vi "ASCII表.vi"() -> ()   [LabVIEW 2012]
uses:
  AsciiCode.ctl
panel:
  out "ASCII（96-127）":string[][](table)
  out "ASCII（64-95）":string[][](table)
  out "ASCII（32-63）":string[][](table)
  out "ASCII（0-31）":string[][](table)
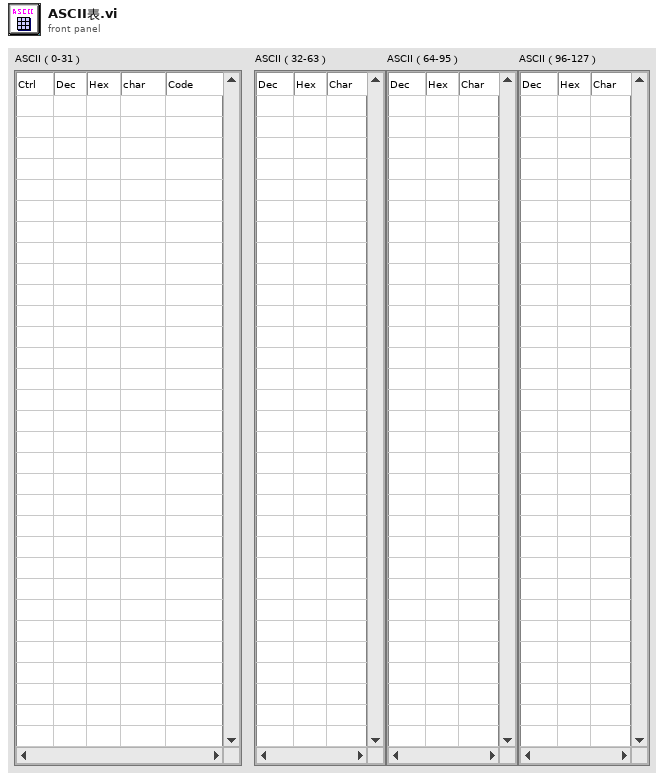
[diagram p1: front panel]
types:
  T1 = typedef "AsciiCode.ctl" = enum16{"NUL", "SOH", "STX", "ETX", "EOT", "ENQ", "ACK", "BEL", "BS", "HT", "LF", "VT", "FF", "CR", "SO", "SI", "DLE", "DC1", "DC2", "DC3", "DC4", "NAK", "SYN", "ETB", "CAN", "EM", "SUB", "ESC", "FS", "GS", "RS", "US"}
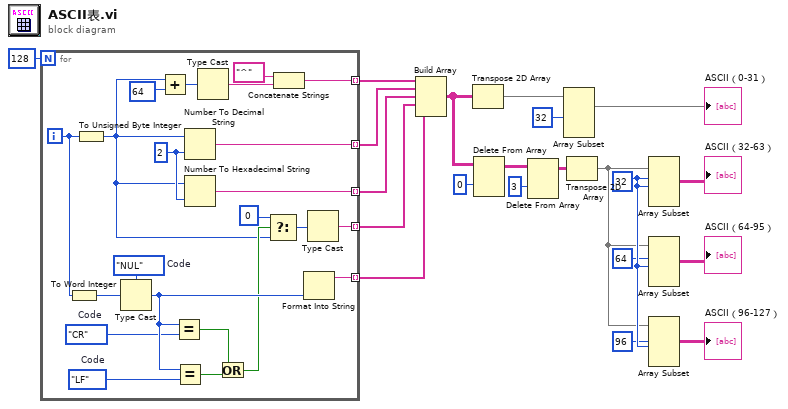
[diagram p0: block diagram]
diagram:
  w6 = 32 ("索引")
  n1 = for {
    N: 128 -> [_]
    tunnel: [w41] -> w20 mode=indexing
    tunnel: [w40] -> w19 mode=indexing
    tunnel: [w39] -> w18 mode=indexing
    tunnel: [w38] -> w16 mode=indexing
    tunnel: [w37] -> w17 mode=indexing
    i -> [w33]
    w23 = i16 2 ("宽度(-)")
    w29 = AsciiCode."CR"  # Code
    w31 = AsciiCode."LF"  # Code
    w42 = AsciiCode."NUL"  # Code
    n2 = To Word Integer(number=w33) -> (16bit integer=w32:i16)
    n3 = To Unsigned Byte Integer(number=w33) -> (unsigned 8bit integer=w22:u8)
    n4 = Type Cast(type=w42, x=w32) -> (*(type *) &x=w30:T1)
    n5 = Add(x=w22, y=u8 64) -> (x+y=w35:u8)
    n6 = Equal?(x=w30, y=w29) -> (x = y?=w27:bool)
    n7 = Equal?(x=w30, y=w31) -> (x = y?=w28:bool)
    n8 = Number To Decimal String(number=w22, width (-)=w23) -> (decimal integer string=w40:string)
    n9 = Number To Hexadecimal String(1:w23, 2:w22) -> (0:w39:string)
    n10 = Type Cast(x=w35) -> (*(type *) &x=w34:string)  [unwired: 1 in]
    n11 = Or(x=w27, y=w28) -> (x .or. y?=w26:bool)
    n12 = Select(t=u8 0 ("y"), s=w26, f=w22) -> (s? t:f=w24:u8)
    n13 = Concatenate Strings("^" ("字符串"), w34) -> (w41:string)
    n14 = Format Into String(w30) -> (resulting string=w38:string)  [unwired: 3 in, 1 out]
    n15 = Type Cast(x=w24) -> (*(type *) &x=w37:string)  [unwired: 1 in]
  }
  n16 = Build Array(w20, w19, w18, w17, w16) -> (w12:string[][])
  n17 = Transpose 2D Array(2D array=w12) -> (transposed array=w13:string[][])
  n18 = Delete From Array(array=w12, index (row)=0 ("长度")) -> (array with subset deleted=w10:string[][])  [unwired: 2 in, 1 out]
  n19 = Delete From Array(array=w10, index (row)=3 ("索引 (行)")) -> (array with subset deleted=w8:string[][])  [unwired: 2 in, 1 out]
  n20 = Array Subset(array=w13, length (row)=32 ("索引")) -> (→"ASCII（0-31）":string[][])  [unwired: 3 in]
  n21 = Transpose 2D Array(2D array=w8) -> (transposed array=w3:string[][])
  n22 = Array Subset(array=w3, index (row)=w6, length (row)=w6) -> (→"ASCII（32-63）":string[][])  [unwired: 2 in]
  n23 = Array Subset(array=w3, index (row)=64 ("索引"), length (row)=w6) -> (→"ASCII（64-95）":string[][])  [unwired: 2 in]
  n24 = Array Subset(array=w3, index (row)=96 ("索引"), length (row)=w6) -> (→"ASCII（96-127）":string[][])  [unwired: 2 in]
